vi "ACQ Status.vi"(8 "error in (no error)":errorcluster, 11 "Conection Data":T1={"VISA resource name"="COM4"}) -> (0 "error out":errorcluster, 3 "Conection Data Out":T1={"VISA resource name"="COM4"})   [LabVIEW 2014, in "SJ-210 Lib.lvlib"]
doc: "Interroga el estado del Rugosimetro y espera hasta que termina de procesar para permitir la salida del VI"
uses:
  SJ-210 Lib.lvlib
  Typedef/Connection Data.ctl
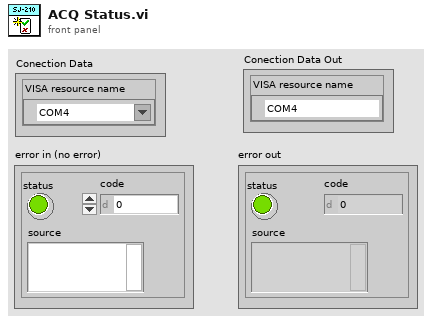
[diagram p1: front panel]
types:
  T1 = typedef "SJ-210 Lib.lvlib/Connection Data.ctl" = cluster{"VISA resource name":refnum<visa-resource-name>}
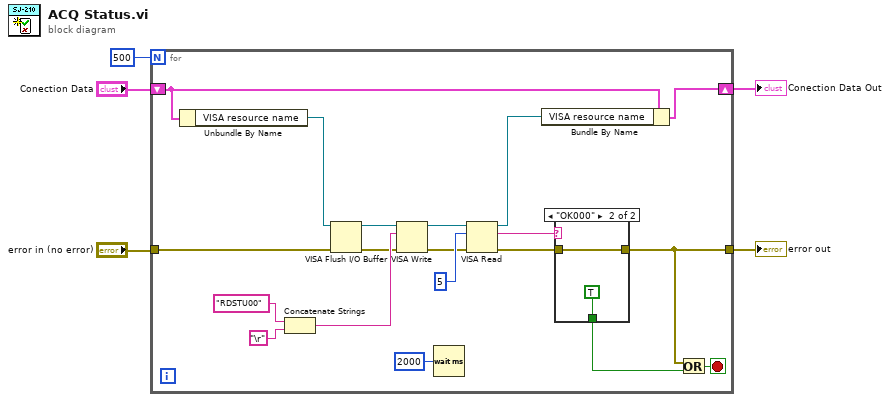
[diagram p0: block diagram]
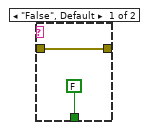
[diagram p2: hidden frame]
diagram:
  n1 = for {
    N: 500 -> [_]
    tunnel: "error in (no error)" -> [w8]
    tunnel: [w6] -> w3
    shift-right: [w19] -> w4
    shift-left: "Conection Data" -> [w20]
    stop <- w14 stop-if-true
    n2 = Unbundle By Name(w20) -> ("VISA resource name"=w9:refnum<visa-resource-name>)
    n3 = Concatenate Strings("RDSTU00" ("write buffer"), "\r") -> (w21:string)
    n4 = VISA Flush I/O Buffer(VISA resource name=w9, error in (no error)=w8) -> (VISA resource name out=w10:refnum<visa-resource-name>, error out=w11:errorcluster)  [unwired: 1 in]
    n5 = VISA Write(VISA resource name=w10, write buffer=w21, error in (no error)=w11) -> (VISA resource name out=w13:refnum<visa-resource-name>, error out=w12:errorcluster)  [unwired: 1 out]
    n6 = Wait (ms)(milliseconds to wait=u32 2000) -> ()  [unwired: 1 out]
    n7 = VISA Read(VISA resource name=w13, byte count=u32 5, error in (no error)=w12) -> (VISA resource name out=w18:refnum<visa-resource-name>, read buffer=w16:string, error out=w7:errorcluster)  [unwired: 1 out]
    n8 = Bundle By Name(cluster=w20, "VISA resource name"=w18) -> (w19:T1)
    n9 = case shown="\"OK000\"" w16 {
      tunnel: [FALSE TRUE] -> w15
      tunnel: w7 -> [w25 w27]
      tunnel: [w25 w27] -> w6
      frame "False", Default {
      }
      frame "OK000" {
      }
    }
    n10 = Or(x=w6, y=w15) -> (x .or. y?=w14:bool)
  }
  "error out" <- w3
  "Conection Data Out" <- w4
